vi "LIDT_PM_UseUSBAddress.vi"(8 "error in (no error)":errorcluster) -> (0 "error out":errorcluster, 1 "OpenDevices":bool, 2 "Output:":string, 3 "new reference":refnum<k24>)   [LabVIEW 2017]
uses:
  C:/Program Files (x86)/Newport/Newport USB Driver/Bin/UsbDllWrap.dll
  Program Files (x86)/Newport/Newport USB Driver/Bin/UsbDllWrap.dll
panel:
  # "Built upon Newport\nUSB Driver v4.2.2"
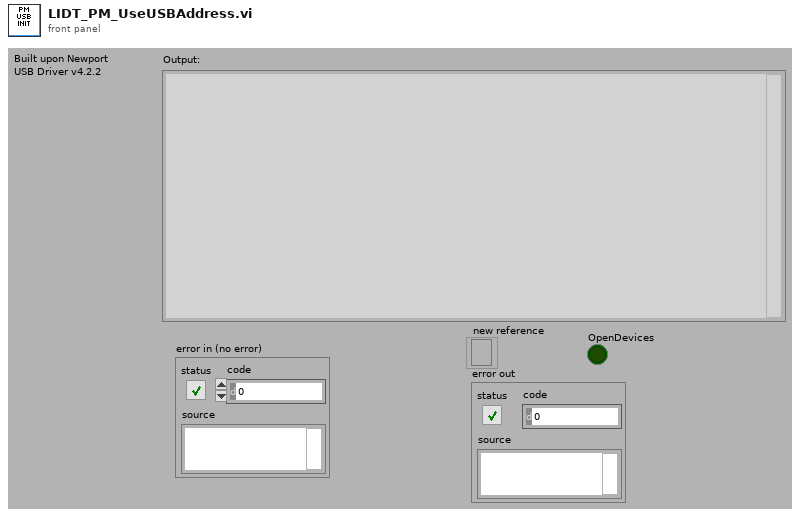
[diagram p1: front panel]
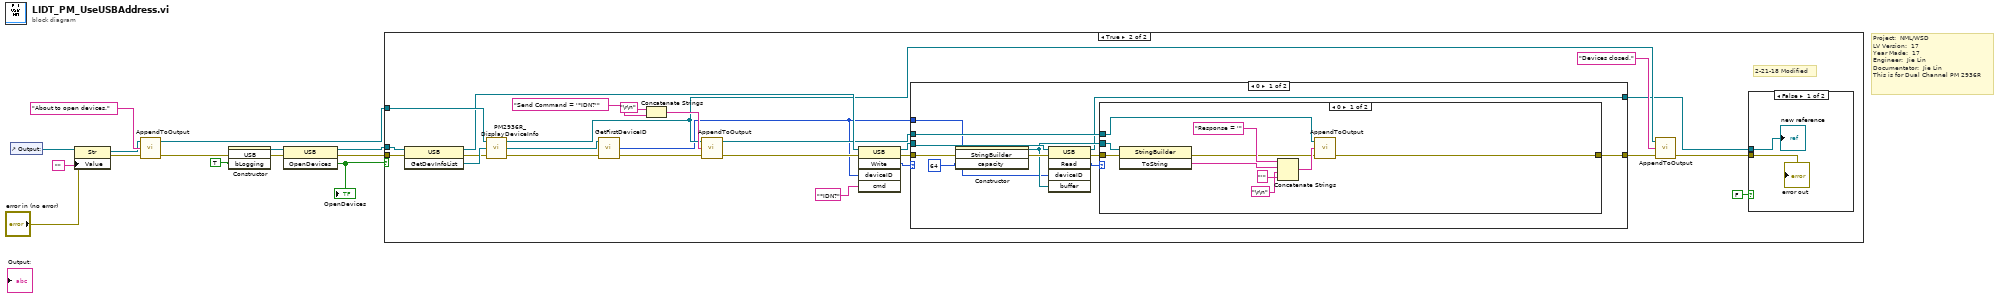
[diagram p0: block diagram]
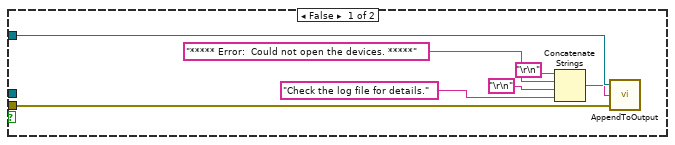
[diagram p2: hidden frame]
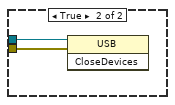
[diagram p3: hidden frame]
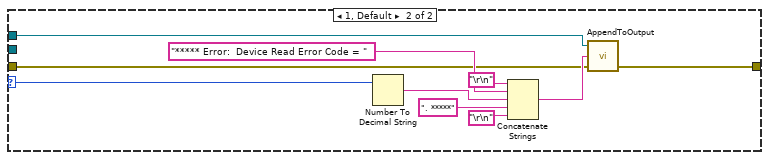
[diagram p4: hidden frame]
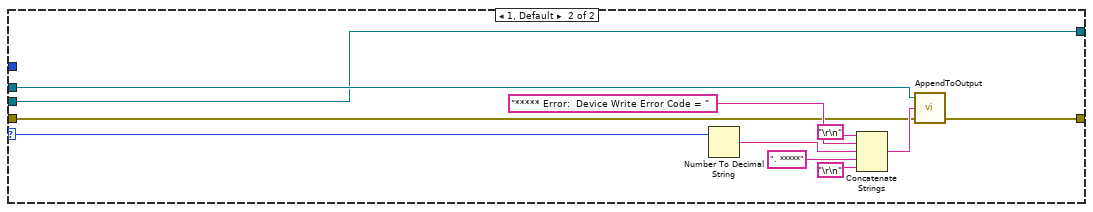
[diagram p5: hidden frame]
diagram:
  # "Project:  NML/WSD \nLV Version:  17\nYear Made:  17\nEngineer:  Jie Lin\nDocumentator:  Jie Lin\nThis is for Dual Channel PM 2936R"
  n1 = control-ref of="Output:"() -> (w5:refnum<vi>)
  n2 = property class="Str"(reference=w5, error in="error in (no error)", "Value"="") -> (reference out=w2:refnum<vi>, error out=w3:errorcluster)
  n3 = call "AppendToOutput.vi"("error in"=w3, "Input String"="About to open devices.", "Output Refnum In"=w2) -> ("error out"=w12:errorcluster, "Output Refnum Out"=w9:refnum<vi>)  [unwired: 1 in]
  n4 = constructor class="USB"(error in=w12, "bLogging"=TRUE) -> (reference out=w11:refnum<k24>, error out=w8:errorcluster)  [unwired: 2 in, 2 out]
  n5 = invoke class="USB" method="OpenDevices"(reference=w11, error in=w8) -> (reference out=w6:refnum<k24>, error out=w7:errorcluster, "OpenDevices"=w10:bool)  [unwired: 1 in]
  "OpenDevices" <- w10
  n6 = case shown="True" w10 {
    tunnel: w9 -> [w21 w44]
    tunnel: w7 -> [w20 w45]
    tunnel: w6 -> [_ w46]
    frame False {
      n7 = Concatenate Strings("\r\n", "***** Error:  Could not open the devices. *****", "\r\n", "Check the log file for details.") -> (w16:string)
      n8 = call "AppendToOutput.vi"("error in"=w20, "Input String"=w16, "Output Refnum In"=w21) -> ()  [unwired: 1 in, 2 out]
    }
    frame True {
      # "2-21-18 Modified"
      n9 = invoke class="USB" method="GetDevInfoList"(reference=w46, error in=w45) -> (reference out=w37:refnum<k24>, error out=w42:errorcluster, "GetDevInfoList"=w43:refnum<k24>)  [unwired: 1 in]
      n10 = call "PM2936R_DisplayDeviceInfo.vi"("error in"=w42, "DevInfoList In"=w43, "Output Refnum In"=w44) -> ("error out"=w35:errorcluster, "DevInfoList Out"=w34:refnum<k24>, "Output Refnum Out"=w27:refnum<vi>)
      n11 = call "GetFirstDeviceID.vi"("error in"=w35, "DevInfoList In"=w34) -> ("error out"=w33:errorcluster, "Device ID"=w25:i32)  [unwired: 1 in, 1 out]
      n12 = Concatenate Strings("\r\n", "Send Command = '*IDN?'") -> (w39:string)
      n13 = call "AppendToOutput.vi"("error in"=w33, "Input String"=w39, "Output Refnum In"=w27) -> ("error out"=w36:errorcluster, "Output Refnum Out"=w29:refnum<vi>)  [unwired: 1 in]
      n14 = invoke class="USB" method="Write"(reference=w37, error in=w36, "deviceID"=w25, "cmd"="*IDN?") -> (reference out=w31:refnum<k24>, error out=w30:errorcluster, "Write"=w32:i32)  [unwired: 1 in, 2 out]
      n15 = case shown="0" w32 {
        selector: w32 -> [_ w87]
        tunnel: w31 -> [w61 w82]
        tunnel: w30 -> [w58 w85]
        tunnel: [w54 w84] -> w26
        tunnel: w29 -> [w53 w83]
        tunnel: w25 -> [w52 _]
        tunnel: [w51 w82] -> w23
        frame 0 {
          n16 = constructor class="StringBuilder"(error in=w58, "capacity"=64) -> (reference out=w56:refnum<k24>, error out=w59:errorcluster)  [unwired: 2 in, 2 out]
          n17 = invoke class="USB" method="Read"(reference=w61, error in=w59, "deviceID"=w52, "buffer"=w56) -> (reference out=w51:refnum<k24>, error out=w55:errorcluster, "Read"=w57:i32)  [unwired: 1 in, 2 out]
          n18 = case shown="0" w57 {
            selector: w57 -> [_ w76]
            tunnel: w56 -> [w71 _]
            tunnel: w55 -> [w70 w73]
            tunnel: [w63 w72] -> w54
            tunnel: w53 -> [w62 w74]
            frame 0 {
              n19 = invoke class="StringBuilder" method="ToString"(reference=w71, error in=w70) -> (error out=w64:errorcluster, "ToString"=w67:string)  [unwired: 1 in, 1 out]
              n20 = Concatenate Strings("Response = '", w67, "'", "\r\n") -> (w65:string)
              n21 = call "AppendToOutput.vi"("error in"=w64, "Input String"=w65, "Output Refnum In"=w62) -> ("error out"=w63:errorcluster)  [unwired: 1 in, 1 out]
            }
            frame 1, Default {
              n22 = Number To Decimal String(number=w76) -> (decimal integer string=w81:string)  [unwired: 1 in]
              n23 = Concatenate Strings("\r\n", "***** Error:  Device Read Error Code = ", w81, ". *****", "\r\n") -> (w75:string)
              n24 = call "AppendToOutput.vi"("error in"=w73, "Input String"=w75, "Output Refnum In"=w74) -> ("error out"=w72:errorcluster)  [unwired: 1 in, 1 out]
            }
          }
        }
        frame 1, Default {
          n25 = Number To Decimal String(number=w87) -> (decimal integer string=w88:string)  [unwired: 1 in]
          n26 = Concatenate Strings("\r\n", "***** Error:  Device Write Error Code = ", w88, ". *****", "\r\n") -> (w86:string)
          n27 = call "AppendToOutput.vi"("error in"=w85, "Input String"=w86, "Output Refnum In"=w83) -> ("error out"=w84:errorcluster)  [unwired: 1 in, 1 out]
        }
      }
      n28 = call "AppendToOutput.vi"("error in"=w26, "Input String"="Devices closed." ("string"), "Output Refnum In"=w27) -> ("error out"=w24:errorcluster)  [unwired: 1 in, 1 out]
      n29 = case shown="False" FALSE {
        tunnel: w24 -> [w47 w50]
        tunnel: w23 -> [w48 w49]
        frame False {
          "new reference" <- w48
          "error out" <- w47
        }
        frame True {
          n30 = invoke class="USB" method="CloseDevices"(reference=w49, error in=w50) -> ()  [unwired: 1 in, 3 out]
        }
      }
    }
  }
